vi "Joystick and Camera.vi"() -> ()   [LabVIEW 2019]
uses:
  Classes/Controller/Camera/Machine Vision.ctl
  Classes/Controller/I-O/I-O.lvclass
  Classes/Controller/Motion/A3200/A3200.lvclass
  Classes/Controller/Camera/Camera.lvclass
  Classes/Controller/Controller.lvclass
panel:
  out "XYZTheta Out":dbl[](array[numeric])
  in  "Machine Vision":T1
  in  "Move 10cm Right":bool
  in  "Move 10cm Backward":bool
  in  "Move 10cm Forward":bool
  in  "Move 10cm Left":bool
  in  "Record Measurement":bool=TRUE
  in  "Dismount Silicon Tray":bool
  in  "Secure Silicon Tray":bool
  in  "Z Go":bool
  in  "Position":dbl
  in  "XYZTheta":dbl[](array[numeric])
  in  "Go":bool
  in  "Joystick":bool
  out "Sum":dbl[](array[numeric])
  out "Gantry":dbl[](array[numeric])
  in  "Stop":bool
  out "Image":T2(plugin-control)
  out "Camera":dbl[](array[numeric])
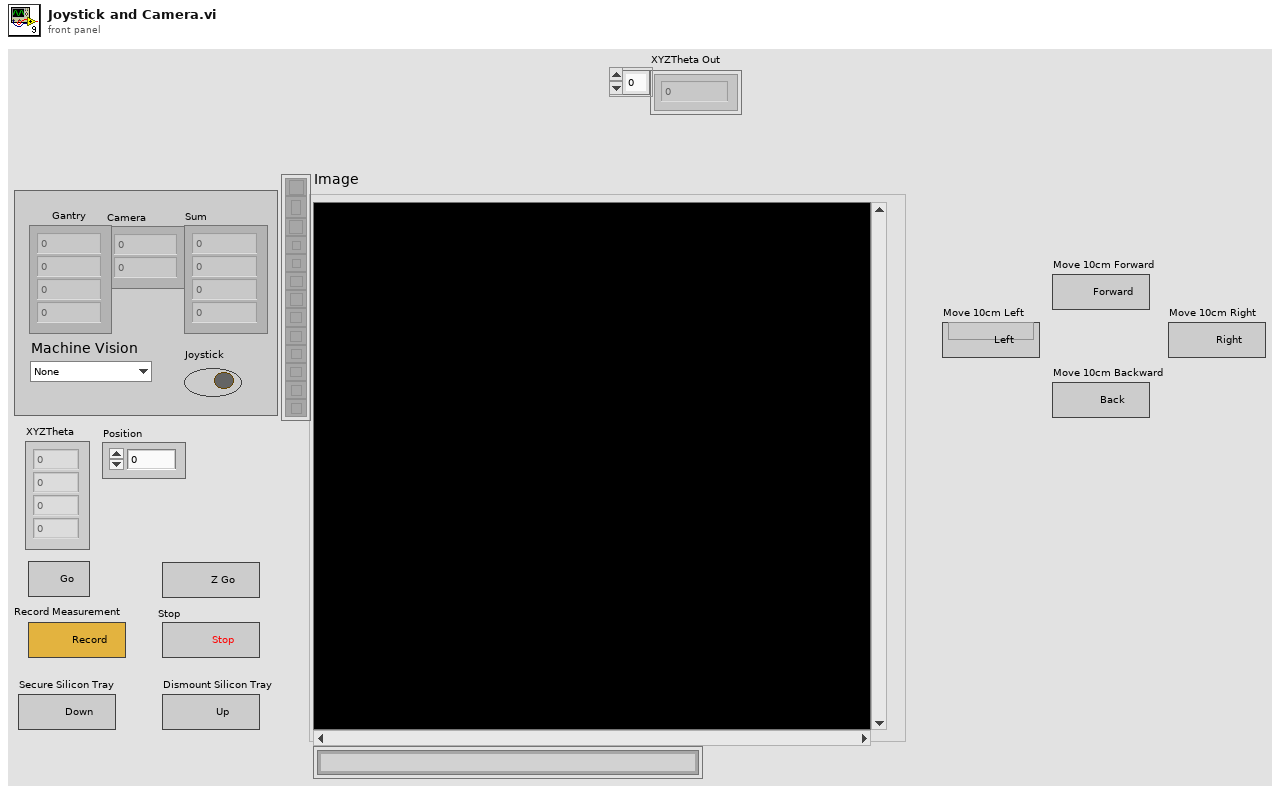
[diagram p1: front panel]
types:
  T1 = typedef "Camera.lvclass/Machine Vision.ctl" = enum16{"None", "Tray Fiducials", "HPK Silicon", "Hexaboard", "Corner (TL, BR)", "Corner (BL, TR)", "silicon top left", "silicon bottom left", "silicon top right", "silicon bottom right", "PCB top left", "PCB bottom left", "PCB top right", "PCB bottom right"}
  T2 = typedef "IMAQ Image.ctl" = refnum<image>
  T3 = enum16{"open", "replace", "create", "open or create", "replace or create", "replace or create with confirmation"}
  T4 = typedef "Controller.lvclass/Controllers.ctl" = cluster{"I-O.lvclass":refnum<class "I-O.lvclass">, "Dispenser.lvclass":refnum<class "Dispenser.lvclass">, "Gantry":refnum<k24>}
  T5 = typedef "I-O.lvclass/Pin Map.ctl" = cluster{"Region Valves":i32[], "Extra Valves":dbl[][][], "Tool Primary Valve":i32, "Tool Secondary Valve":i32, "Region Sensors":i32[], "Extra Sensors":dbl[][][], "Tool Primary Sensor":dbl, "Tool Secondary Sensor":dbl, "Compression Sensor":dbl, "5V":i32}
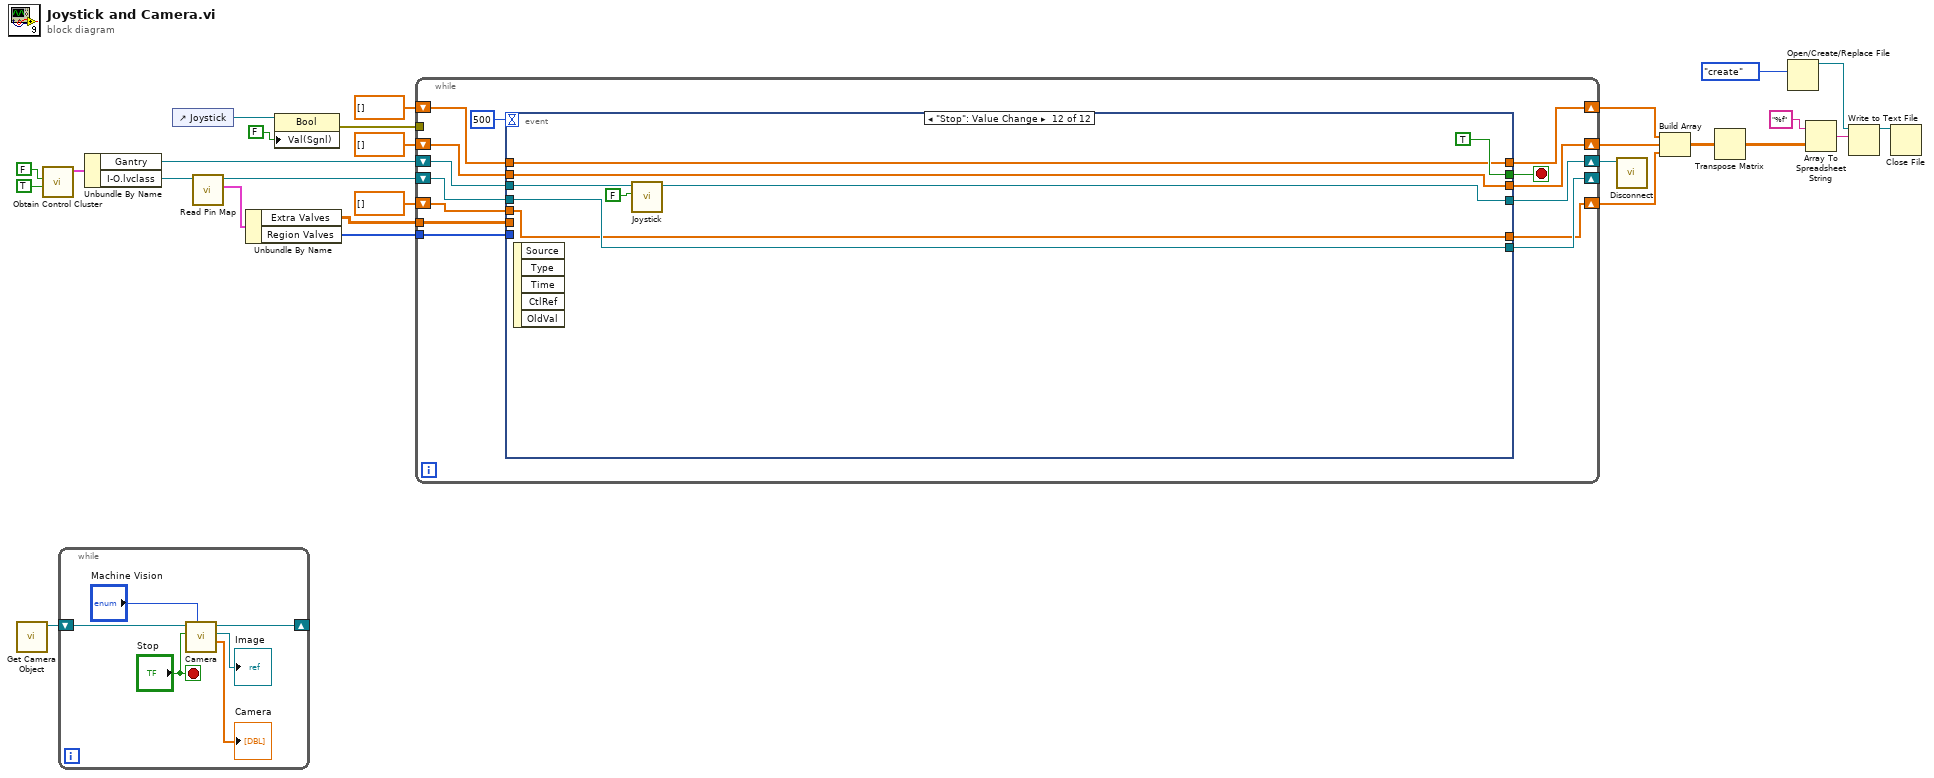
[diagram p0: block diagram]
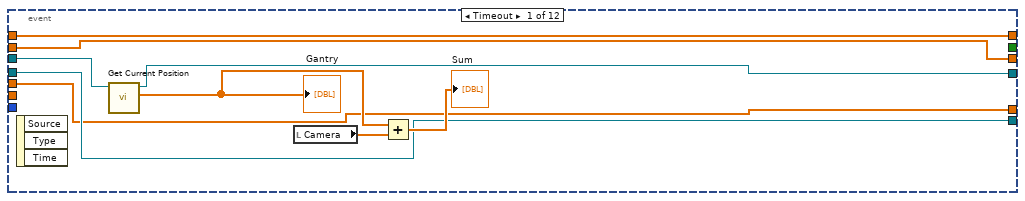
[diagram p2: hidden frame]
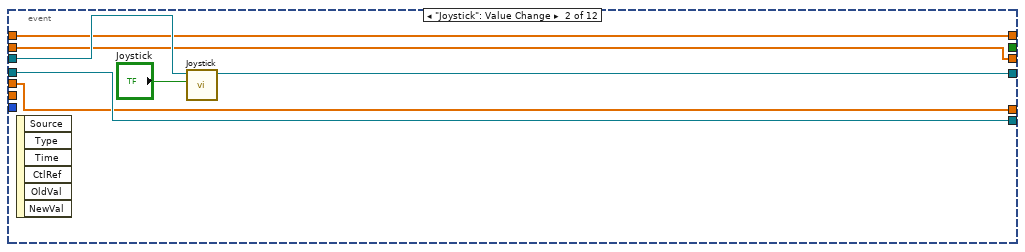
[diagram p3: hidden frame]
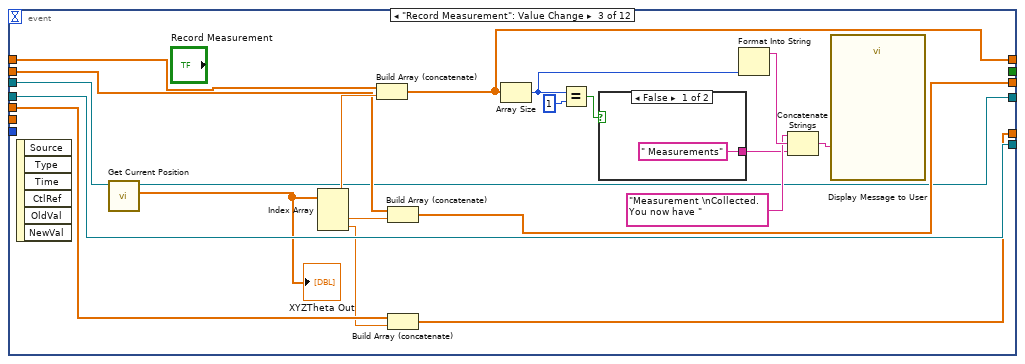
[diagram p4: hidden frame]
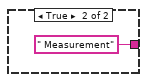
[diagram p5: hidden frame]
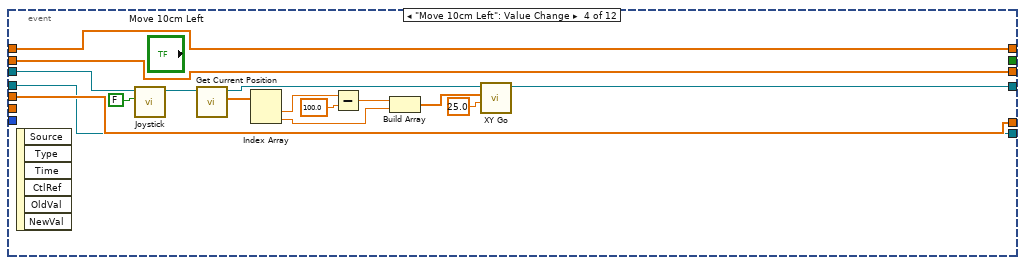
[diagram p6: hidden frame]
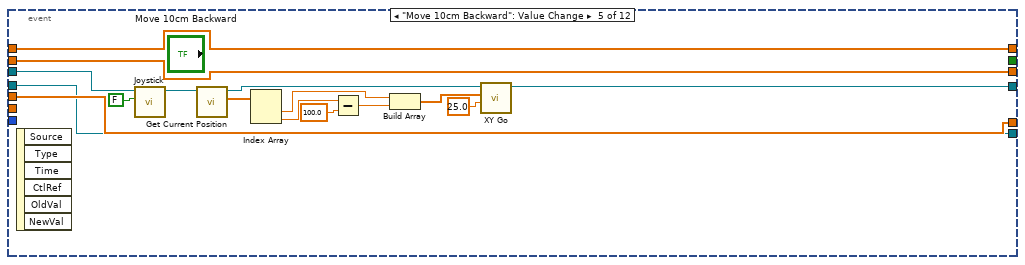
[diagram p7: hidden frame]
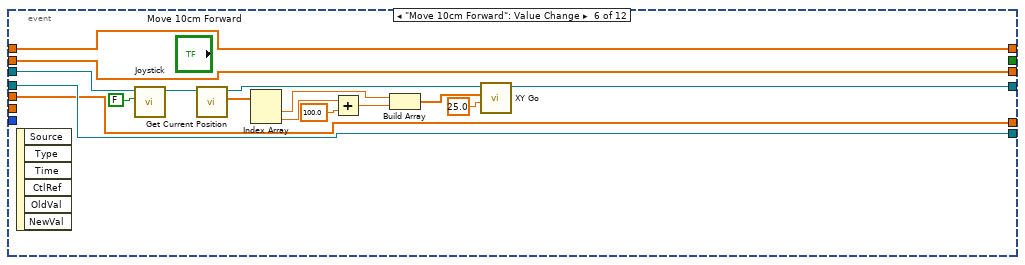
[diagram p8: hidden frame]
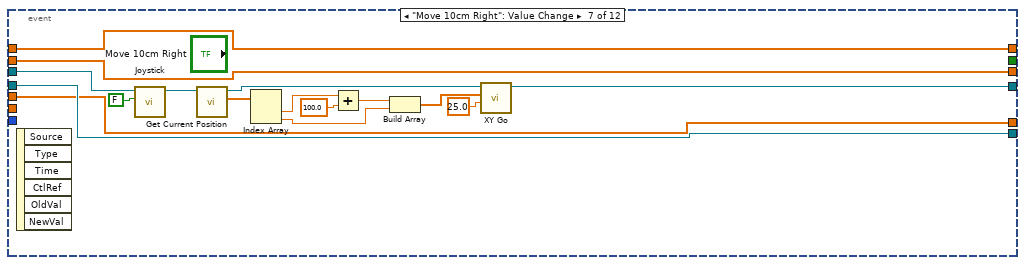
[diagram p9: hidden frame]
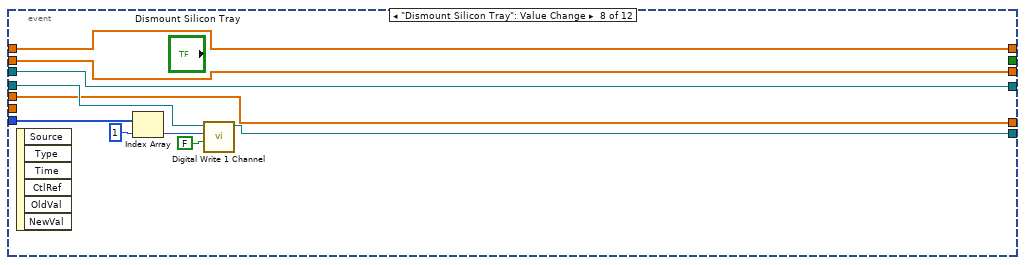
[diagram p10: hidden frame]
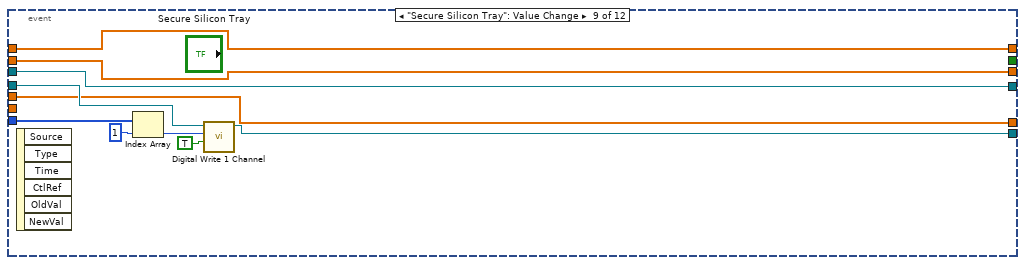
[diagram p11: hidden frame]
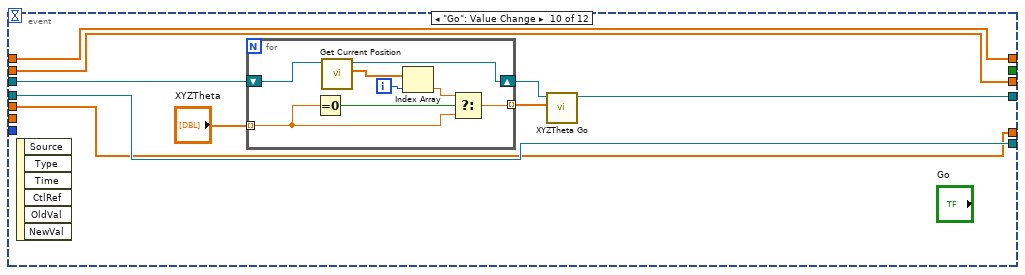
[diagram p12: hidden frame]
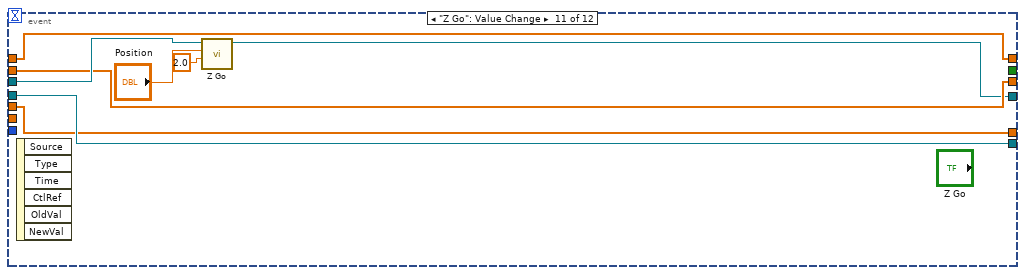
[diagram p13: hidden frame]
diagram:
  n1 = call "Get Camera Object.vi"() -> ("Camera out"=w19:refnum<class "Camera.lvclass">)  [unwired: 10 in, 1 out]
  n2 = call "Obtain Control Cluster.vi"("I/O"=TRUE, "Dispense"=FALSE) -> ("Control Out"=w21:T4)  [unwired: 9 in]
  n3 = while {
    shift-right: [w32] -> _
    shift-left: w19 -> [w33]
    stop <- "Stop" stop-if-true
    n4 = call "Camera.vi"("Machine Vision"="Machine Vision", "Stop"="Stop", "Camera in"=w33) -> ("Camera"=→"Camera":dbl[], "Image"=→"Image":T2, "Camera out"=w32:refnum<class "Camera.lvclass">)  [unwired: 5 in, 1 out]
  }
  n5 = Unbundle By Name(w21) -> ("Gantry"=w20:refnum<k24>, "I-O.lvclass"=w18:refnum<class "I-O.lvclass">)
  n6 = control-ref of="Joystick"() -> (w26:refnum<vi>)
  n7 = call-dynamic "Read Pin Map.vi"("I-O in"=w18) -> ("Pin Map 2"=w16:T5, "I-O out"=w17:refnum<class "I-O.lvclass">)  [unwired: 8 in, 1 out]
  n8 = Unbundle By Name(w16) -> ("Extra Valves"=w14:dbl[][][], "Region Valves"=w15:i32[])
  n9 = property class="Bool"(reference=w26, "Val(Sgnl)"=FALSE ("Value (Signaling)")) -> (error out=w24:errorcluster)  [unwired: 1 in, 1 out]
  n10 = while {
    shift-right: [w34] -> w25
    shift-left: w20 -> [w45]
    tunnel: w24 -> [_]
    shift-right: [w43] -> _
    shift-left: w17 -> [w44]
    tunnel: w15 -> [w42]
    tunnel: w14 -> [w41]
    shift-right: [w36] -> w2
    shift-left: dbl[] [] -> [w40]
    shift-right: [w38] -> w3
    shift-left: dbl[] [] -> [w39]
    shift-right: [w35] -> w4
    shift-left: dbl[] [] -> [w37]
    stop <- w46 stop-if-true
    n11 = event shown="[11] \"Stop\": Value Change" {
      selector: _ -> [_ _ _ _ _ _ _ _ _ _ _ _]
      dyn-events: _ -> [_ _ _ _ _ _ _ _ _ _ _ _]
      timeout: 500 -> [_ _ _ _ _ _ _ _ _ _ _ _]
      tunnel: [_ _ _ _ _ _ _ _ _ _ _ TRUE] -> w46
      tunnel: w45 -> [w54 w63 w83 w93 w108 w124 w140 w150 w160 w177 w194 w201]
      tunnel: w44 -> [w53 w61 w82 w87 w103 w120 w136 w157 w169 w174 w191 w199]
      tunnel: [w53 w61 w82 w87 w103 w120 w136 w154 w164 w174 w191 w199] -> w43
      tunnel: w42 -> [_ _ _ _ _ _ _ w159 w168 _ _ _]
      tunnel: w41 -> [_ _ _ _ _ _ _ _ _ _ _ _]
      tunnel: w40 -> [w51 w60 w68 w90 w106 w122 w138 w153 w163 w173 w190 w198]
      tunnel: [w51 w60 w72 w90 w106 w122 w138 w153 w163 w173 w190 w198] -> w36
      tunnel: w39 -> [w50 w59 w69 w89 w105 w121 w137 w152 w162 w172 w189 w197]
      tunnel: [w50 w59 w71 w89 w105 w121 w137 w152 w162 w172 w189 w197] -> w38
      tunnel: w37 -> [w49 w58 w67 w88 w104 w119 w135 w151 w161 w171 w188 w196]
      tunnel: [w49 w58 w65 w88 w104 w119 w135 w151 w161 w171 w188 w196] -> w35
      tunnel: [w48 w57 w64 w86 w102 w118 w134 w150 w160 w170 w187 w195] -> w34
      event Timeout {
        n12 = event-data() -> ()  [unwired: 1 in, 3 out]
        n13 = call "Get Current Position.vi"("Gantry In"=w54) -> ("XYZTheta Out"=w52:dbl[], "Gantry Out"=w48:refnum<k24>)  [unwired: 8 in, 1 out]
        "Gantry" <- w52
        n14 = local read "Camera"() -> (w56:dbl[])
        n15 = Add(x=w52, y=w56) -> (x+y=→"Sum":dbl[])
      }
      event "Joystick": Value Change {
        n16 = event-data() -> ()  [unwired: 1 in, 6 out]
        n17 = call "Joystick.vi"("Joystick"="Joystick", "Gantry In"=w63) -> ("Gantry Out"=w57:refnum<k24>)  [unwired: 8 in, 1 out]
      }
      event "Record Measurement": Value Change {
        n18 = event-data() -> ()  [unwired: 1 in, 6 out]
        n19 = call "Get Current Position.vi"("Gantry In"=w83) -> ("XYZTheta Out"=w73:dbl[], "Gantry Out"=w64:refnum<k24>)  [unwired: 8 in, 1 out]
        "XYZTheta Out" <- w73
        n20 = Index Array(array=w73) -> (element #1=w81:dbl, element #2=w70:dbl, element #3=w66:dbl)  [unwired: 3 in]
        n21 = Build Array (concatenate) "Build Array"(w69, w81) -> (w71:dbl[])
        n22 = Build Array (concatenate)(w68, w70) -> (w72:dbl[])
        n23 = Build Array (concatenate)(w67, w66) -> (w65:dbl[])
        n24 = Array Size(array=w71) -> (size(s)=w76:i32)
        n25 = Equal?(x=w76, y=1) -> (x = y?=w75:bool)
        n26 = case shown="False" w75 {
          tunnel: [" Measurements" " Measurement"] -> w74
          frame False {
          }
          frame True {
          }
        }
        n27 = Format Into String(w76) -> (resulting string=w80:string)  [unwired: 3 in, 1 out]
        n28 = Concatenate Strings("Measurement \nCollected. You now have ", w80, w74) -> (w78:string)
        n29 = call "Display Message to User"("Message"=w78) -> ()  [unwired: 9 in, 2 out]
      }
      event "Move 10cm Left": Value Change {
        n30 = event-data() -> ()  [unwired: 1 in, 6 out]
        n31 = call "Joystick.vi"("Joystick"=FALSE, "Gantry In"=w93) -> ("Gantry Out"=w92:refnum<k24>)  [unwired: 8 in, 1 out]
        n32 = call "Get Current Position.vi"("Gantry In"=w92) -> ("XYZTheta Out"=w100:dbl[], "Gantry Out"=w101:refnum<k24>)  [unwired: 8 in, 1 out]
        n33 = Index Array(array=w100) -> (element #1=w99:dbl, element #2=w96:dbl)  [unwired: 2 in]
        n34 = Subtract(x=w99, y=100.0) -> (x-y=w97:dbl)
        n35 = Build Array(w97, w96) -> (w95:dbl[])
        n36 = call "XY Go.vi"("Speed"=25.0, "XY"=w95, "Gantry In"=w101) -> ("Gantry Out"=w86:refnum<k24>)  [unwired: 7 in, 1 out]
      }
      event "Move 10cm Backward": Value Change {
        n37 = event-data() -> ()  [unwired: 1 in, 6 out]
        n38 = call "Joystick.vi"("Joystick"=FALSE, "Gantry In"=w108) -> ("Gantry Out"=w107:refnum<k24>)  [unwired: 8 in, 1 out]
        n39 = call "Get Current Position.vi"("Gantry In"=w107) -> ("XYZTheta Out"=w116:dbl[], "Gantry Out"=w117:refnum<k24>)  [unwired: 8 in, 1 out]
        n40 = Index Array(array=w116) -> (element #1=w111:dbl, element #2=w114:dbl)  [unwired: 2 in]
        n41 = Subtract(x=w114, y=100.0) -> (x-y=w112:dbl)
        n42 = Build Array(w111, w112) -> (w110:dbl[])
        n43 = call "XY Go.vi"("Speed"=25.0, "XY"=w110, "Gantry In"=w117) -> ("Gantry Out"=w102:refnum<k24>)  [unwired: 7 in, 1 out]
      }
      event "Move 10cm Forward": Value Change {
        n44 = event-data() -> ()  [unwired: 1 in, 6 out]
        n45 = call "Joystick.vi"("Joystick"=FALSE, "Gantry In"=w124) -> ("Gantry Out"=w123:refnum<k24>)  [unwired: 8 in, 1 out]
        n46 = call "Get Current Position.vi"("Gantry In"=w123) -> ("XYZTheta Out"=w132:dbl[], "Gantry Out"=w133:refnum<k24>)  [unwired: 8 in, 1 out]
        n47 = Index Array(array=w132) -> (element #1=w127:dbl, element #2=w128:dbl)  [unwired: 2 in]
        n48 = Add(x=w128, y=100.0) -> (x+y=w126:dbl)
        n49 = Build Array(w127, w126) -> (w130:dbl[])
        n50 = call "XY Go.vi"("Speed"=25.0, "XY"=w130, "Gantry In"=w133) -> ("Gantry Out"=w118:refnum<k24>)  [unwired: 7 in, 1 out]
      }
      event "Move 10cm Right": Value Change {
        n51 = event-data() -> ()  [unwired: 1 in, 6 out]
        n52 = call "Joystick.vi"("Joystick"=FALSE, "Gantry In"=w140) -> ("Gantry Out"=w139:refnum<k24>)  [unwired: 8 in, 1 out]
        n53 = call "Get Current Position.vi"("Gantry In"=w139) -> ("XYZTheta Out"=w148:dbl[], "Gantry Out"=w149:refnum<k24>)  [unwired: 8 in, 1 out]
        n54 = Index Array(array=w148) -> (element #1=w142:dbl, element #2=w145:dbl)  [unwired: 2 in]
        n55 = Add(x=w142, y=100.0) -> (x+y=w146:dbl)
        n56 = Build Array(w146, w145) -> (w144:dbl[])
        n57 = call "XY Go.vi"("Speed"=25.0, "XY"=w144, "Gantry In"=w149) -> ("Gantry Out"=w134:refnum<k24>)  [unwired: 7 in, 1 out]
      }
      event "Dismount Silicon Tray": Value Change {
        n58 = event-data() -> ()  [unwired: 1 in, 6 out]
        n59 = Index Array(array=w159, index=1) -> (element=w156:i32)
        n60 = call-dynamic "Digital Write 1 Channel.vi"("Value"=FALSE, "Channel"=w156, "I-O.lvclass"=w157) -> ("I-O.lvclass 2"=w154:refnum<class "I-O.lvclass">)  [unwired: 7 in, 1 out]
      }
      event "Secure Silicon Tray": Value Change {
        n61 = event-data() -> ()  [unwired: 1 in, 6 out]
        n62 = Index Array(array=w168, index=1) -> (element=w166:i32)
        n63 = call-dynamic "Digital Write 1 Channel.vi"("Value"=TRUE, "Channel"=w166, "I-O.lvclass"=w169) -> ("I-O.lvclass 2"=w164:refnum<class "I-O.lvclass">)  [unwired: 7 in, 1 out]
      }
      event "Go": Value Change {
        n64 = event-data() -> ()  [unwired: 1 in, 6 out]
        n65 = for {
          tunnel: "XYZTheta" -> [w184] mode=indexing
          tunnel: [w182] -> w176 mode=indexing
          shift-right: [w180] -> w175
          shift-left: w177 -> [w181]
          i -> [w186]
          n66 = Equal To 0?(x=w184) -> (x = 0?=w185:bool)
          n67 = call "Get Current Position.vi"("Gantry In"=w181) -> ("XYZTheta Out"=w179:dbl[], "Gantry Out"=w180:refnum<k24>)  [unwired: 8 in, 1 out]
          n68 = Index Array(array=w179, index=w186) -> (element=w183:dbl)
          n69 = Select(t=w183, s=w185, f=w184) -> (s? t:f=w182:dbl)
        }
        n70 = call "XYZTheta Go.vi"("XYZTheta In"=w176, "Gantry In"=w175) -> ("Gantry Out"=w170:refnum<k24>)  [unwired: 7 in, 2 out]
      }
      event "Z Go": Value Change {
        n71 = event-data() -> ()  [unwired: 1 in, 6 out]
        n72 = call "Z Go.vi"("Speed"=2.0, "Position"="Position", "Gantry In"=w194) -> ("Gantry Out"=w187:refnum<k24>)  [unwired: 7 in, 1 out]
      }
      event "Stop": Value Change {
        n73 = event-data() -> ()  [unwired: 1 in, 5 out]
        n74 = call "Joystick.vi"("Joystick"=FALSE, "Gantry In"=w201) -> ("Gantry Out"=w195:refnum<k24>)  [unwired: 8 in, 1 out]
      }
    }
  }
  n75 = call "Disconnect.vi"("Gantry In"=w25) -> ()  [unwired: 9 in, 1 out]
  n76 = Build Array(w3, w2, w4) -> (w8:dbl[][])
  n77 = Transpose Matrix(1:w8) -> (0:w7:dbl[][])
  n78 = Open/Create/Replace File(operation (0:open)=T3."create") -> (refnum out=w6:refnum<file>)  [unwired: 5 in, 2 out]
  n79 = Array To Spreadsheet String(array=w7, 3:"%f" ("format string")) -> (spreadsheet string=w10:string)  [unwired: 1 in]
  n80 = Write to Text File(file (use dialog)=w6, text=w10) -> (refnum out=w9:refnum<file>)  [unwired: 2 in, 2 out]
  n81 = Close File(refnum=w9) -> ()  [unwired: 1 in, 2 out]
